vi "亂數產生.vi"() -> ()   [LabVIEW 2015]
panel:
  out "Waveform Chart":T1(graph)
  in  "Boolean":bool
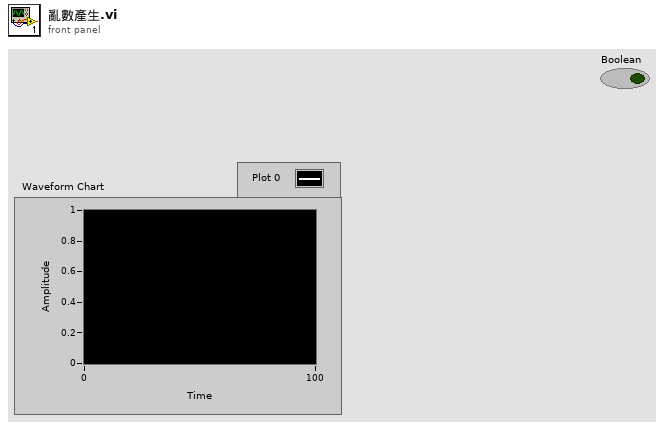
[diagram p1: front panel]
types:
  T1 = cluster{"number: 0 to 1":dbl, "number: 0 to 1":dbl, "element":dbl}
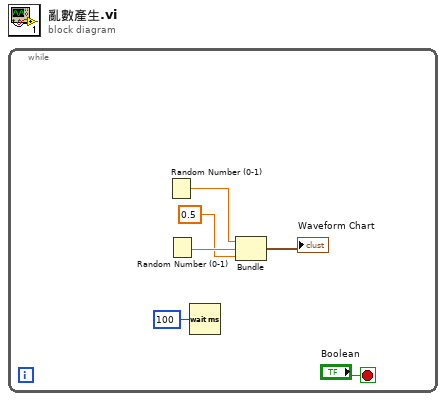
[diagram p0: block diagram]
diagram:
  n1 = while {
    stop <- "Boolean" stop-if-true
    n2 = Random Number (0-1)() -> (number: 0 to 1=w4:dbl)
    n3 = Random Number (0-1)() -> (number: 0 to 1=w3:dbl)
    n4 = Wait (ms)(milliseconds to wait=u32 100) -> ()  [unwired: 1 out]
    n5 = Bundle("number: 0 to 1"=w4, "number: 0 to 1"=w3, "element"=0.5) -> (→"Waveform Chart":T1)  [unwired: 1 in]
  }
